vi "decimalAdd.vi"(8 "Error In":errorcluster, 10 "Frequency/PWM%":string, 11 "refnum in":refnum<file>) -> (0 "error out":errorcluster, 2 "concatenated string":string, 3 "refnum out":refnum<file>)   [LabVIEW 2018]
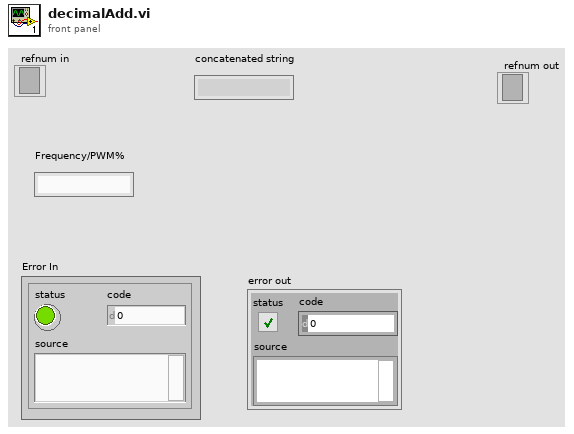
[diagram p1: front panel]
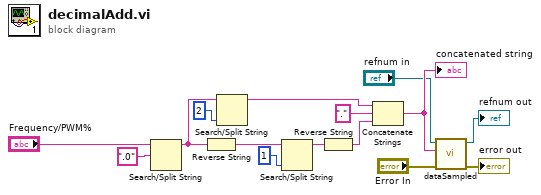
[diagram p0: block diagram]
diagram:
  n1 = Search/Split String(string="Frequency/PWM%", search string/char (-)=".0") -> (substring before match=w12:string)  [unwired: 1 in, 2 out]
  n2 = Reverse String(1:w12) -> (0:w11:string)
  n3 = Search/Split String(string=w12, offset (0)=2) -> (substring before match=w7:string)  [unwired: 1 in, 2 out]
  n4 = Search/Split String(string=w11, offset (0)=1) -> (substring before match=w14:string)  [unwired: 1 in, 2 out]
  n5 = Reverse String(1:w14) -> (0:w6:string)
  n6 = Concatenate Strings(w7, "." ("string"), w6) -> (w5:string)
  "concatenated string" <- w5
  n7 = call "dataSampled.vi"("Error In"="Error In", "Data"=w5, "refnum in"="refnum in") -> ("error out"=→"error out":errorcluster, "refnum out"=→"refnum out":refnum<file>)  [unwired: 7 in]
